vi "Write NET_WebProxy.vi"(8 "error in (no error)":errorcluster, 10 "NET_WebProxy":refnum<k24>, 11 "WebProxy_NET in":refnum<class "WebProxy_NET.lvclass">) -> (0 "error out":errorcluster, 3 "WebProxy_NET out":refnum<class "WebProxy_NET.lvclass">)   [LabVIEW 2018, in "HttpClient_NET.lvlib" / "WebProxy_NET.lvclass"]
doc: "<b> </b> <b> </b>\nHttpClient_NET\nJustin Young - Viviota\nCopyright (c) 2021\nLicense: BSD"
uses:
  WebProxy_NET.lvclass
  WebProxy_NET.lvclass/WebProxy_NET.ctl
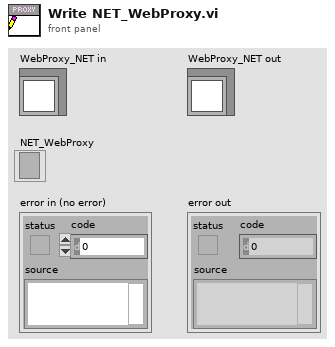
[diagram p1: front panel]
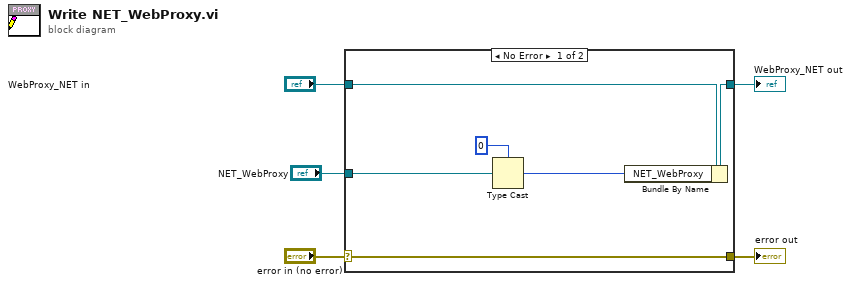
[diagram p0: block diagram]
diagram:
  n1 = case shown="No Error" "error in (no error)" {
    selector: "error in (no error)" -> [w11 w12]
    tunnel: [w11 w12] -> w4
    tunnel: [w9 w13] -> w2
    tunnel: "WebProxy_NET in" -> [w10 w13]
    tunnel: "NET_WebProxy" -> [w8 _]
    frame No Error {
      n2 = Type Cast(type=i64 0 ("NET_WebProxy"), x=w8) -> (*(type *) &x=w6:i64)
      n3 = Bundle By Name(cluster=w10, "NET_WebProxy"=w6) -> (w9:refnum<class "WebProxy_NET.lvclass">)
    }
    frame Error {
    }
  }
  "error out" <- w4
  "WebProxy_NET out" <- w2
